vi "TPNPT_AverageSamples.vi"(0 "Values":dbl[](array[numeric]) format="%.2f", 1 "last value":dbl format="%.2f", 2 "Number of samples":i32, 4 "index":i32) -> (7 "average":dbl format="%.2f", 8 "Values out":dbl[](array[numeric]) format="%.2f")   [LabVIEW 2016]
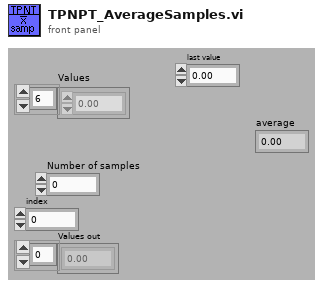
[diagram p1: front panel]
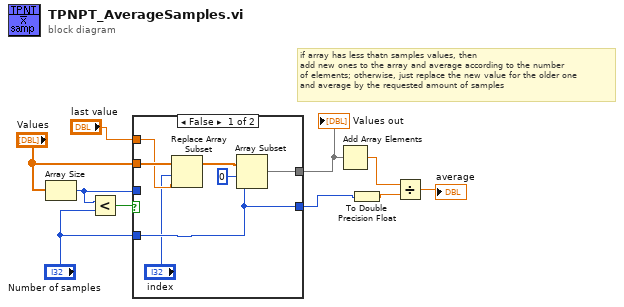
[diagram p0: block diagram]
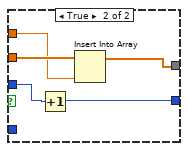
[diagram p2: hidden frame]
diagram:
  # "if array has less thatn samples values, then\nadd new ones to the array and average according to the number\nof elements; otherwise, just replace the new value for the older one\nand average by the requested amount of samples"
  n1 = Array Size(array="Values") -> (size(s)=w1:i32)
  n2 = Less?(x=w1, y="Number of samples") -> (x < y?=w3:bool)
  n3 = case shown="False" w3 {
    tunnel: [w16 w20] -> w10
    tunnel: "Values" -> [w14 w22]
    tunnel: [w15 w18] -> w5
    tunnel: "Number of samples" -> [w15 _]
    tunnel: "last value" -> [w12 w21]
    tunnel: w1 -> [_ w19]
    frame False {
      n4 = Replace Array Subset(array=w14, new element=w12, index="index") -> (w13:dbl[])
      n5 = Array Subset(array=w13, index=0 ("Array Index"), length=w15) -> (w16:dbl[])
    }
    frame True {
      n6 = Increment(x=w19) -> (x+1=w18:i32)
      n7 = Insert Into Array(array=w22, new element=w21) -> (w20:dbl[])  [unwired: 1 in]
    }
  }
  "Values out" <- w10
  n8 = Add Array Elements(numeric array=w10) -> (sum=w9:dbl)
  n9 = To Double Precision Float(number=w5) -> (double precision float=w8:dbl)
  n10 = Divide(x=w9, y=w8) -> (x/y=→"average":dbl)
